vi "NT Read and Format Entries as Tree.vi"(6 "Tags to  Close":string[](array[string]), 8 "error in":errorcluster, 9 "Operation":enum16{"Update", "Clear"}(ring), 10 "Name Pattern":string, 11 "Tree Refnum":refnum<vi>) -> (0 "error out":errorcluster, 3 "Formatted Strings":cluster{"Name":string, "Value":string}[](array[cluster]))   [LabVIEW 2017]
doc: "Retrieve the entries that match the name pattern, and use the / seperators to construct the tree. Provide the reference to the tree control that you would like to be updated, or use the name/value pairs to update your own list, table, etc. Supported wildcards are * and ?."
uses:
  <vilib>/Rock Robotics/Network Tables/Make Table Operation.ctl
panel:
  in  "Tree":string(tree)
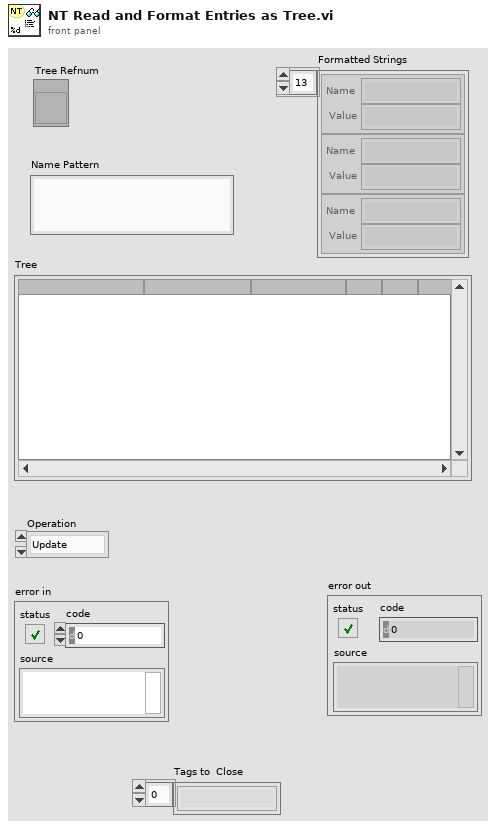
[diagram p1: front panel]
types:
  T1 = cluster{"Left Cell String":string, "Child Text":string[], "Child Tag":string, "Item Indent":i32, "Child Only?":bool, "Glyph Index":i32}[]
  T2 = typedef "Make Table Operation.ctl" = enum16{"Get or Add Field", "Get Field or Add Temp", "Replace Temp ID", "Get Field ID - No Add", "Get Table Field IDs", "Get Field ID Info", "Move Field to Temp", "Validate", "Remove Field", "Remove All"}
  T3 = cluster{"Left Cell String":string, "Child Text":string[], "Child Tag":string, "Item Indent":i32, "Child Only?":bool, "Glyph Index":i32}
  T4 = typedef "Field ID.ctl" = i32
  T5 = typedef "Field Data.ctl" = cluster{"Dbl":dbl, "String":string, "Type":T6, "Boolean":bool, "Sequence #":T7, "Flags":u8}
  T6 = typedef "Field Type.ctl" = enum8{"Invalid", "Bool", "Numeric", "String", "Raw", "Boolean Array", "Numeric Array", "String Array", "RPC"}
  T7 = typedef "Sequence.ctl" = u16
  T8 = cluster{"Left Cell String":bool, "Child Text":bool[], "Child Tag":bool, "Item Indent":bool, "Child Only?":bool, "Glyph Index":bool}[]
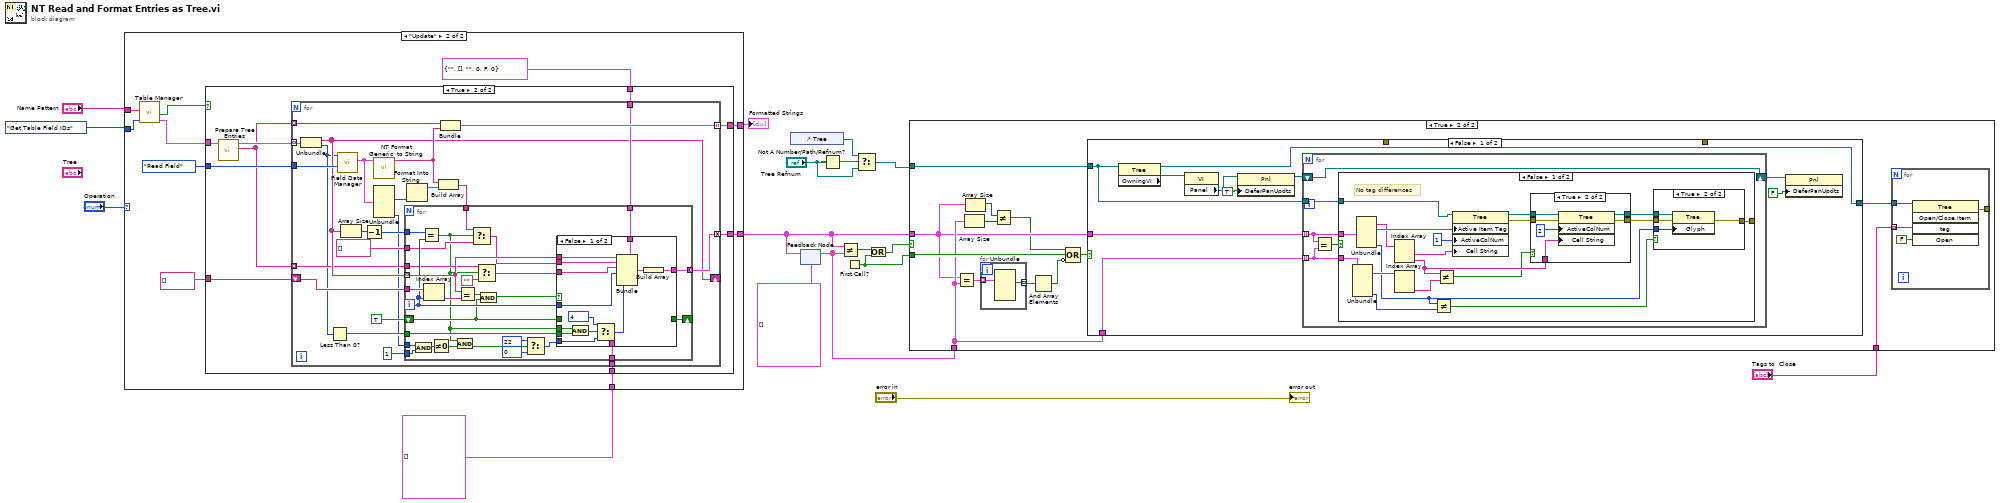
[diagram p0: block diagram]
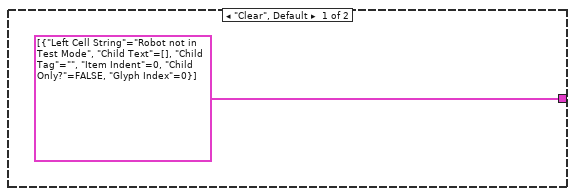
[diagram p2: hidden frame]
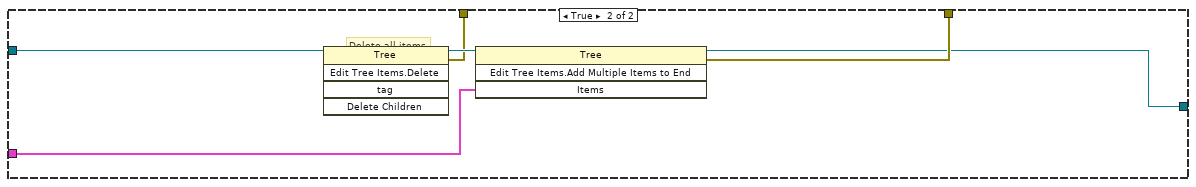
[diagram p9: hidden frame]
diagram:
  n1 = case shown="\"Update\"" "Operation" {
    tunnel: [_ w28] -> w17
    tunnel: Make_Table_Operation."Get Table Field IDs" ("Operation") -> [_ w26]
    tunnel: "Name Pattern" -> [_ w23]
    tunnel: T1 [] -> [_ w21]
    tunnel: [T1 [{"Left Cell String"="Robot not in Test Mode", "Child Text"=[], "Child Tag"="", "Item Indent"=0, "Child Only?"=FALSE, "Glyph Index"=0}] w19] -> w8
    frame "Clear", Default {
    }
    frame "Update" {
      n2 = call <vilib>:"Table Manager.vi"("Operation"=w26, "Entry Name"=w23) -> ("Entries"=w22:cluster{"Entry IDs":T4[], "Names":string[]}, "Success"=w24:bool)  [unwired: 6 in, 2 out]
      n3 = case shown="True" w24 {
        tunnel: [_ w37] -> w28
        tunnel: enum16{"Update Field", "Read Field"}."Read Field" ("Operation") -> [_ w36]
        tunnel: [_ w35] -> w19
        tunnel: T3 {"Left Cell String"="", "Child Text"=[], "Child Tag"="", "Item Indent"=0, "Child Only?"=FALSE, "Glyph Index"=0} ("Item") -> [_ w34]
        tunnel: string[] [] ("Child Text") -> [_ w33]
        tunnel: w22 -> [_ w30]
        tunnel: w21 -> [_ w31]
        frame False {
        }
        frame True {
          n4 = call <vilib>:"Prepare Tree Entries.vi"("Entries"=w30) -> ("Tokens"=w29:string[], "Sorted Tree Rows"=w32:cluster{"Array":string[], "Field ID":T4}[])  [unwired: 9 in]
          n5 = for {
            tunnel: [w59] -> w37 mode=indexing
            tunnel: w36 -> [w60]
            tunnel: [w49] -> w35 mode=concatenating
            tunnel: w34 -> [w50]
            shift-right: [w44] -> _
            shift-left: w33 -> [w52]
            tunnel: w29 -> [w54] mode=indexing
            tunnel: w32 -> [w53] mode=indexing
            tunnel: w31 -> [w51]
            tunnel: w29 -> [w43] mode=indexing
            n6 = Unbundle(w53) -> ("Array"=w44:string[], "Field ID"=w41:T4)
            n7 = Less Than 0?(x=w41) -> (x < 0?=w40:bool)
            n8 = call <vilib>:"Field Data Manager.vi"("Operation"=w60, "Field ID"=w41) -> ("Field Value Out"=w57:T5)  [unwired: 8 in, 1 out]
            n9 = Array Size(array=w44) -> (size(s)=w48:i32)
            n10 = Decrement(x=w48) -> (x-1=w47:i32)
            n11 = call <vilib>:"NT Format Generic  to String.vi"("Field Value"=w57) -> ("String"=w58:string)  [unwired: 10 in]
            n12 = Unbundle(w57) -> ("Type"=w55:T6, "Flags"=w39:u8)  [unwired: 4 out]
            n13 = Format Into String(w55) -> (resulting string=w56:string)  [unwired: 3 in, 1 out]
            n14 = Build Array(w58, w56) -> (w46:string[])
            n15 = for {
              tunnel: w52 -> [w88]
              tunnel: w44 -> [w83] mode=indexing
              tunnel: w51 -> [w86]
              tunnel: [w85] -> w49 mode=concatenating
              tunnel: w50 -> [w84]
              tunnel: w47 -> [w81]
              tunnel: w46 -> [w80]
              tunnel: string[] [] ("appended array") -> [w78]
              tunnel: w43 -> [w76]
              shift-right: [w72] -> _
              shift-left: TRUE -> [w71]
              tunnel: w40 -> [w70]
              tunnel: w39 -> [w66]
              tunnel: u8 1 -> [w65]
              i -> [w82]
              n16 = Compound Arithmetic op=AND(w66, w65) -> (w64:u8)
              n17 = Equal?(x=w81, y=w82) -> (x = y?=w61:bool)
              n18 = Index Array(array=w88, index=w82) -> (element=w87:string)
              n19 = Not Equal To 0?(x=w64) -> (x != 0?=w63:bool)
              n20 = Equal?(x=w83, y=w87) -> (x = y?=w74:bool)
              n21 = Compound Arithmetic op=AND(w61, w63) -> (w62:bool)
              n22 = Select(t=w80, s=w61, f=w78) -> (s? t:f=w79:string[])
              n23 = Select(t=w76, s=w61, f="") -> (s? t:f=w77:string)
              n24 = And(x=w74, y=w71) -> (x .and. y?=w73:bool)
              n25 = Select(t=22, s=w62, f=0) -> (s? t:f=w69:i32)
              n26 = case shown="False" w73 {
                tunnel: [w99 w103] -> w85
                tunnel: w86 -> [_ w103]
                tunnel: w84 -> [w101 _]
                tunnel: w83 -> [w98 _]
                tunnel: w82 -> [w97 _]
                tunnel: w79 -> [w96 _]
                tunnel: w77 -> [w95 _]
                tunnel: [_ w102] -> w72
                tunnel: w71 -> [_ w102]
                tunnel: w61 -> [w94 _]
                tunnel: w70 -> [w93 _]
                tunnel: w69 -> [w90 _]
                frame False {
                  n27 = And(x=w94, y=w93) -> (x .and. y?=w92:bool)
                  n28 = Select(t=4, s=w92, f=w90) -> (s? t:f=w89:i32)
                  n29 = Bundle(cluster=w101, "Left Cell String"=w98, "Child Text"=w96, "Child Tag"=w95, "Item Indent"=w97, "Glyph Index"=w89) -> (w100:T3)  [unwired: 1 in]
                  n30 = Build Array(w100) -> (w99:T1)
                }
                frame True {
                }
              }
            }
            n31 = Bundle(w54, "String"=w58) -> (w59:cluster{string, "String":string})  [unwired: 1 in]
          }
        }
      }
    }
  }
  "Formatted Strings" <- w17
  n32 = control-ref of="Tree"() -> (w14:refnum<vi>)
  n33 = feedback-in #1(w8) -> ()
  n34 = feedback #1(T1 []) -> (w2:T1)
  n35 = Not A Number/Path/Refnum?(number/path/refnum="Tree Refnum") -> (NaN/Path/Refnum?=w15:bool)
  n36 = Not Equal?(x=w8, y=w2) -> (x != y?=w6:bool)
  n37 = First Call?() -> (First Call?: T/F=w3:bool)
  n38 = Select(t=w14, s=w15, f="Tree Refnum") -> (s? t:f=w4:refnum<vi>)
  n39 = Or(x=w6, y=w3) -> (x .or. y?=w7:bool)
  n40 = case shown="True" w7 {
    tunnel: w4 -> [_ w116]
    tunnel: w8 -> [_ w109]
    tunnel: w3 -> [_ w114]
    tunnel: w2 -> [_ w110]
    tunnel: "Tags to  Close" -> [_ w105]
    frame False {
    }
    frame True {
      n41 = Equal?(x=w109, y=w110) -> (x = y?=w111:T8)
      n42 = Array Size(array=w110) -> (size(s)=w108:i32)
      n43 = Array Size(array=w109) -> (size(s)=w107:i32)
      n44 = for {
        tunnel: w111 -> [w122] mode=indexing
        tunnel: [w121] -> w115 mode=indexing
        n45 = Unbundle(w122) -> ("Child Tag"=w121:bool)  [unwired: 5 out]
      }
      n46 = Not Equal?(x=w107, y=w108) -> (x != y?=w106:bool)
      n47 = And Array Elements(Boolean array=w115) -> (logical AND=w113:bool)
      n48 = Compound Arithmetic op=OR(w106, w114, invert w113) -> (w112:bool)
      n49 = case shown="False" w112 {
        tunnel: w116 -> [w130 w174]
        tunnel: w109 -> [w132 w171]
        tunnel: w110 -> [w131 _]
        tunnel: [_ w173] -> _
        tunnel: [_ w172] -> _
        tunnel: [w123 w170] -> w104
        frame False {
          n50 = property class="Tree"(reference=w130) -> (reference out=w123:refnum<vi>, "OwningVI"=w129:refnum<vi>)  [unwired: 1 in, 1 out]
          n51 = property class="VI"(reference=w129) -> ("Panel"=w128:refnum<vi>)  [unwired: 1 in, 2 out]
          n52 = property class="Pnl"(reference=w128, "DeferPanUpdts"=TRUE) -> (reference out=w126:refnum<vi>)  [unwired: 1 in, 1 out]
          n53 = for {
            tunnel: w132 -> [w136] mode=indexing
            tunnel: w131 -> [w135] mode=indexing
            tunnel: w130 -> [w134]
            shift-right: [w133] -> w124
            shift-left: w126 -> [w133]
            n54 = Equal?(x=w136, y=w135) -> (x = y?=w137:bool)
            n55 = case shown="False" w137 {
              tunnel: w136 -> [w156 _]
              tunnel: w135 -> [w145 _]
              tunnel: w134 -> [w152 _]
              tunnel: [w147 _] -> _
              frame False {
                # "No tag differences"
                n56 = Unbundle(w145) -> ("Child Text"=w144:string[], "Glyph Index"=w139:i32)  [unwired: 4 out]
                n57 = Unbundle(w156) -> ("Child Text"=w146:string[], "Child Tag"=w155:string, "Glyph Index"=w140:i32)  [unwired: 3 out]
                n58 = Index Array(array=w146) -> (element #1=w153:string, element #2=w142:string)  [unwired: 2 in]
                n59 = Index Array(array=w144) -> (element #2=w143:string)  [unwired: 2 in, 1 out]
                n60 = Not Equal?(x=w140, y=w139) -> (x != y?=w138:bool)
                n61 = Not Equal?(x=w142, y=w143) -> (x != y?=w141:bool)
                n62 = property class="Tree"(reference=w152, "Active Item Tag"=w155, "ActiveColNum"=1 ("Active Cell:Active Column Number"), "Cell String"=w153) -> (reference out=w149:refnum<vi>, error out=w151:errorcluster)  [unwired: 1 in]
                n63 = case shown="True" w141 {
                  tunnel: w151 -> [w162 w169]
                  tunnel: [w162 w168] -> w150
                  tunnel: w149 -> [w163 w167]
                  tunnel: [w163 w166] -> w148
                  tunnel: w142 -> [_ w164]
                  frame False {
                  }
                  frame True {
                    n64 = property class="Tree"(reference=w167, error in=w169, "ActiveColNum"=2 ("Active Cell:Active Column Number"), "Cell String"=w164) -> (reference out=w166:refnum<vi>, error out=w168:errorcluster)
                  }
                }
                n65 = case shown="True" w138 {
                  tunnel: w150 -> [w157 w161]
                  tunnel: w148 -> [_ w160]
                  tunnel: [w157 w159] -> w147
                  tunnel: w140 -> [_ w158]
                  frame False {
                  }
                  frame True {
                    n66 = property class="Tree"(reference=w160, error in=w161, "Glyph"=w158) -> (error out=w159:errorcluster)  [unwired: 1 out]
                  }
                }
              }
              frame True {
              }
            }
          }
          n67 = property class="Pnl"(reference=w124, "DeferPanUpdts"=FALSE) -> ()  [unwired: 1 in, 2 out]
        }
        frame True {
          # "Delete all items"
          n68 = invoke class="Tree" method="Edit Tree Items.Delete"(reference=w174) -> (reference out=w175:refnum<vi>, error out=w173:errorcluster)  [unwired: 4 in, 3 out]
          n69 = invoke class="Tree" method="Edit Tree Items.Add Multiple Items to End"(reference=w175, "Items"=w171) -> (reference out=w170:refnum<vi>, error out=w172:errorcluster)  [unwired: 2 in, 2 out]
        }
      }
      n70 = for {
        tunnel: w105 -> [w119] mode=indexing
        tunnel: w104 -> [w120]
        tunnel: [w117] -> _
        n71 = invoke class="Tree" method="Open/Close.Item"(reference=w120, "tag"=w119, "Open"=FALSE ("Open?")) -> (error out=w117:errorcluster)  [unwired: 2 in, 4 out]
      }
    }
  }
  "error out" <- "error in"
